vi "Delete Range DVR.vi"(8 "error in (no error)":errorcluster, 11 "Range DVR in":refnum<data-value>) -> (0 "error out":errorcluster, 3 "Range out":refnum<class "Range.lvclass">)   [LabVIEW 2012, in "MDSplus.lvlib" / "Range.lvclass"]
uses:
  <vilib>/MDSplus/Classes/Data_Class/Compound_Class/Range_Class/Range.lvclass
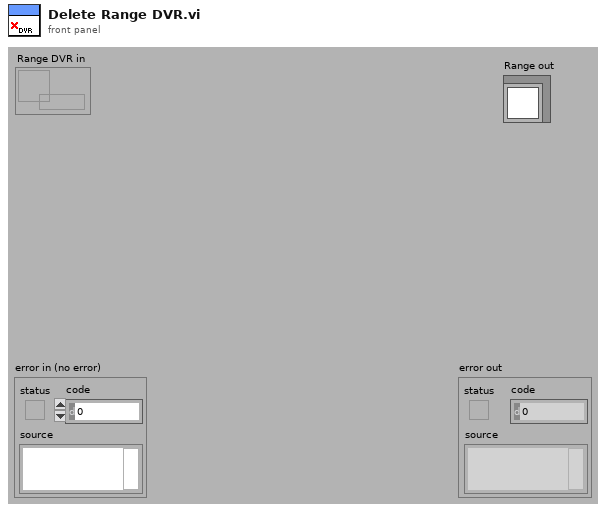
[diagram p1: front panel]
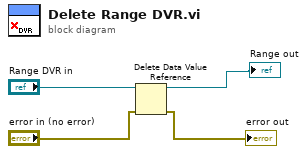
[diagram p0: block diagram]
diagram:
  n1 = Delete Data Value Reference(data value reference="Range DVR in", error in="error in (no error)") -> (data value=→"Range out":refnum<class "Range.lvclass">, error out=→"error out":errorcluster)
